vi "FL_Get_Zone_presence_time.vi"(1 "Present in Zone":bool) -> (0 "Zone presence time, s":dbl)   [LabVIEW 2018, in "Tracker.lvlib"]
uses:
  Tracker.lvlib
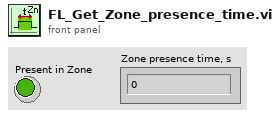
[diagram p1: front panel]
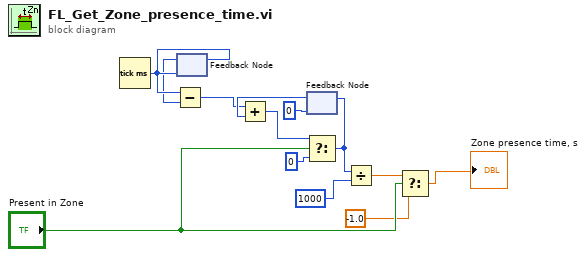
[diagram p0: block diagram]
diagram:
  n1 = Tick Count (ms)() -> (millisecond timer value=w7:u32)
  n2 = feedback #1(w7) -> (w6:u32)
  n3 = Subtract(x=w7, y=w6) -> (x-y=w8:u32)
  n4 = feedback-in #1(w7) -> ()
  n5 = feedback #2(u32 0) -> (w9:u32)
  n6 = Add(x=w8, y=w9) -> (x+y=w11:u32)
  n7 = Select(t=w11, s="Present in Zone", f=u32 0) -> (s? t:f=w13:u32)
  n8 = feedback-in #2(w13) -> ()
  n9 = Divide(x=w13, y=u32 1000) -> (x/y=w4:dbl)
  n10 = Select(t=w4, s="Present in Zone", f=-1.0) -> (s? t:f=→"Zone presence time, s":dbl)
